vi "Log Debug Event.vi"(8 "error in (no error)":errorcluster, 10 "Debug Data.lvclass":refnum<class "Debug Data.lvclass">, 11 "Debugger in":refnum<class "Debug Log.lvclass">) -> (0 "error out":errorcluster, 3 "Debugger out":refnum<class "Debug Log.lvclass">)   [LabVIEW 2020, in "Debug Log.lvclass"]
uses:
  Debug Log.lvclass
  Debug Data/Debug Data.lvclass
  Debug Data/Debug Data.lvclass/Debug Data.ctl
  Debug Log.lvclass/Debug Log.ctl
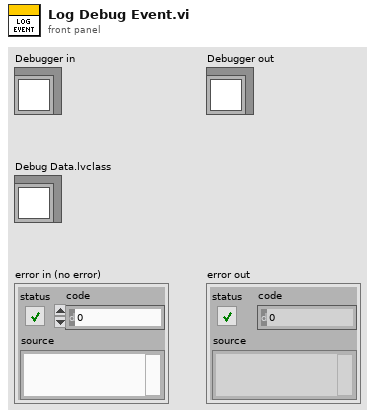
[diagram p1: front panel]
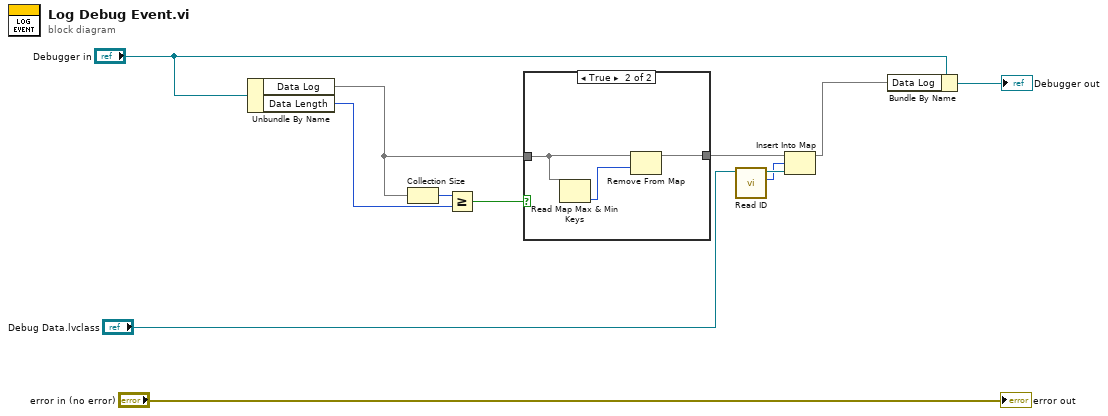
[diagram p0: block diagram]
diagram:
  n1 = Unbundle By Name("Debugger in") -> ("Data Log"=w5:map{u32, refnum<class "Debug Data.lvclass">}, "Data Length"=w7:i32)
  n2 = Collection Size(1:w5) -> (0:w8:i32)
  n3 = Greater Or Equal?(x=w8, y=w7) -> (x >= y?=w6:bool)
  n4 = case shown="True" w6 {
    tunnel: w5 -> [w13 w16]
    tunnel: [w13 w14] -> w4
    frame False {
    }
    frame True {
      n5 = Read Map Max & Min Keys(11:w16) -> (1:w15:u32)  [unwired: 1 out]
      n6 = Remove From Map(10:w15, 11:w16) -> (3:w14:map{u32, refnum<class "Debug Data.lvclass">})  [unwired: 2 out]
    }
  }
  n7 = call "Read ID.vi"("Debug Data in"="Debug Data.lvclass") -> ("ID"=w2:u32, "Debug Data out"=w3:refnum<class "Debug Data.lvclass">)  [unwired: 8 in, 1 out]
  n8 = Insert Into Map(map in=w4, key=w2, value=w3) -> (map out=w1:map{u32, refnum<class "Debug Data.lvclass">})  [unwired: 2 out]
  n9 = Bundle By Name(cluster="Debugger in", "Data Log"=w1) -> (→"Debugger out":refnum<class "Debug Log.lvclass">)
  "error out" <- "error in (no error)"
